vi "Group Publishing.vi"() -> ()   [LabVIEW 2020, in "VectoScratch.lvlib"]
uses:
  VectoScratch.lvlib
  Vecto/Group Info.ctl
  Vecto/Publish Config.ctl
  Vecto/Channel Init.ctl
  4d34a514-e5b9-4f11-b735-09902ffeac7b.vi
  Vecto/ChannelService/ChannelService.lvclass
  Vecto/RemoteDataService/RemoteDataService.lvclass
  Vecto/Vecto.lvlib
  Vecto/Group Config/Group Config.lvclass
  Vecto/Group/Group.lvclass
  Vecto/SequenceCountService/SequenceCountService.lvclass
panel:
  in  "Groups":i32=100
  in  "Rate":i32=10
  in  "Count":i32=150
  out "error out":errorcluster
  out "i":i32
  in  "stop":bool
  in  "Publish Address":string="230.0.0.100"
  in  "Publish Port":u16=20000
  in  "Node Name":string="Alpha"
  in  "Values":dbl[][](array[slide]) scale=0.0..1000.0
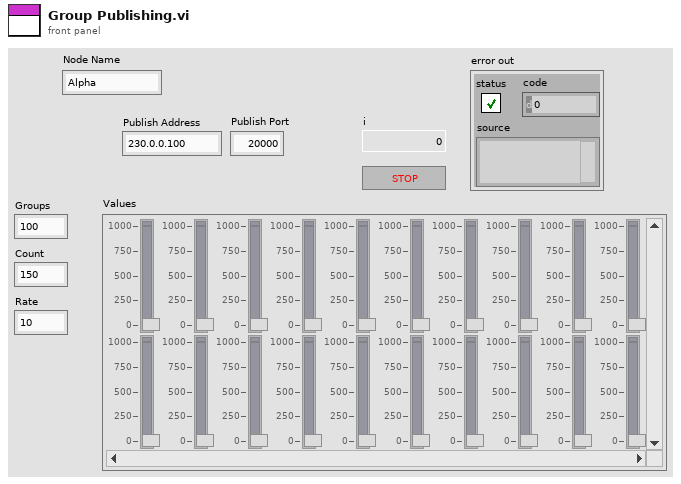
[diagram p1: front panel]
types:
  T1 = typedef "Vecto.lvlib/Publish Config.ctl" = cluster{"Address":string, "Port":u16}
  T2 = typedef "Vecto.lvlib/Group Info.ctl" = cluster{"System":string, "Cluster":string, "Node":string, "Task":string, "Name":string}
  T3 = typedef "Vecto.lvlib/Channel Init.ctl" = cluster{"Name":string, "Resource":string}
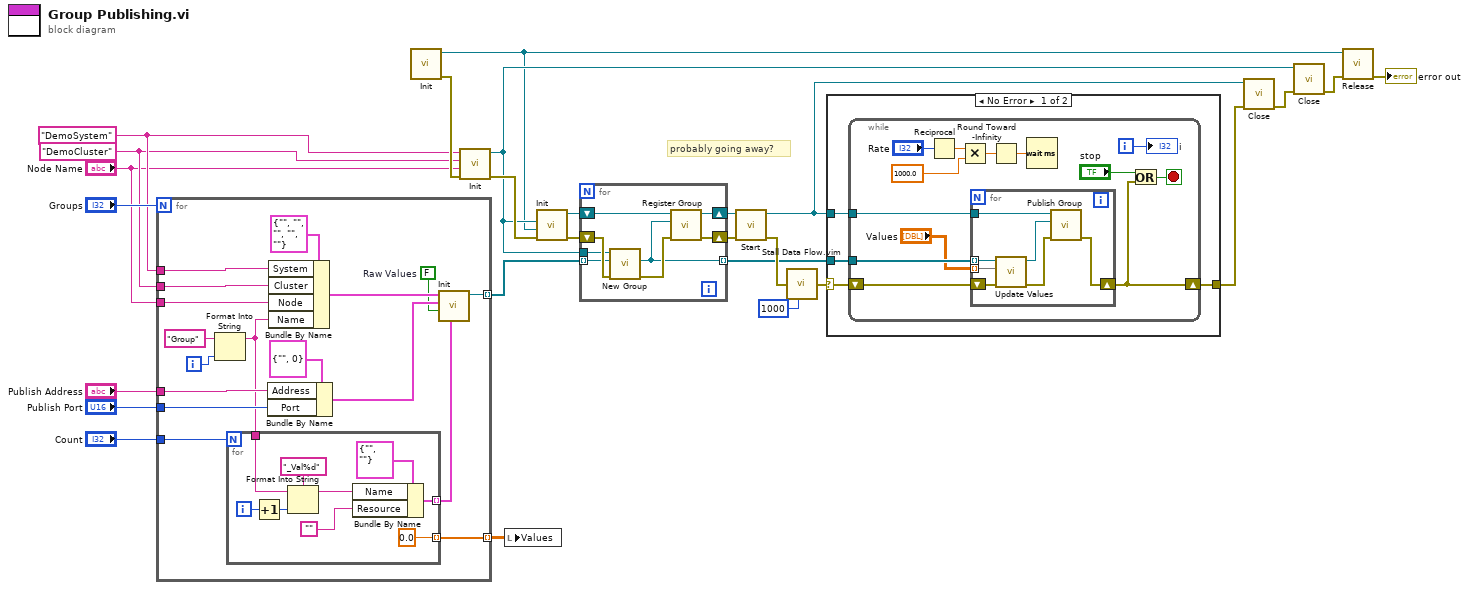
[diagram p0: block diagram]
diagram:
  w14 = "DemoSystem" ("System")
  w13 = "DemoCluster" ("Cluster")
  # "probably going away?"
  n1 = for {
    N: "Groups" -> [_]
    tunnel: w14 -> [w42]
    tunnel: w13 -> [w41]
    tunnel: "Node Name" -> [w40]
    tunnel: "Publish Address" -> [w38]
    tunnel: "Publish Port" -> [w37]
    tunnel: [w32] -> w21 mode=indexing
    tunnel: [w31] -> w20 mode=indexing
    tunnel: "Count" -> [w30]
    i -> [w28]
    w33 = FALSE  # Raw Values
    n2 = Format Into String(initial string="Group", w28) -> (resulting string=w27:string)  [unwired: 2 in, 1 out]
    n3 = for {
      N: w30 -> [_]
      tunnel: [w45] -> w34 mode=indexing
      tunnel: [0.0] -> w31 mode=indexing
      tunnel: w27 -> [w46]
      i -> [w52]
      n4 = Increment(x=w52) -> (x+1=w51:i32)
      n5 = Format Into String(format string="_Val%d", initial string=w46, w51) -> (resulting string=w49:string)  [unwired: 1 in, 1 out]
      n6 = Bundle By Name(cluster=T3 {"Name"="", "Resource"=""} ("Channel Init"), "Name"=w49, "Resource"="") -> (w45:T3)
    }
    n7 = Bundle By Name(cluster=T1 {"Address"="", "Port"=0} ("Publish Config"), "Address"=w38, "Port"=w37) -> (w35:T1)
    n8 = Bundle By Name(cluster=T2 {"System"="", "Cluster"="", "Node"="", "Task"="", "Name"=""} ("Group Info"), "System"=w42, "Cluster"=w41, "Node"=w40, "Name"=w27) -> (w36:T2)
    n9 = call "Init.vi"("Channels"=w34, "Raw Values (T)"=w33, "Publish Config (None)"=w35, "Group Info"=w36) -> ("Group Config out"=w32:refnum<class "Group Config.lvclass">)  [unwired: 6 in, 1 out]
  }
  n10 = call "Init.vi"() -> ("error out"=w24:errorcluster, "SequenceCountService out"=w2:refnum<class "SequenceCountService.lvclass">)  [unwired: 10 in]
  n11 = call "Init.vi"("error in (no error)"=w24, "Node"="Node Name", "Cluster"=w13, "System"=w14) -> ("error out"=w25:errorcluster, "ChannelService out"=w4:refnum<class "ChannelService.lvclass">)  [unwired: 6 in]
  n12 = local write "Values"(w20) -> ()
  n13 = call "Init.vi"("error in (no error)"=w25, "SequenceCountService"=w2, "ChannelService"=w4) -> ("error out"=w10:errorcluster, "RemoteDataService out"=w11:refnum<class "RemoteDataService.lvclass">)  [unwired: 7 in]
  n14 = for {
    tunnel: w4 -> [w58]
    tunnel: w21 -> [w54] mode=indexing
    tunnel: [w53] -> w17 mode=indexing
    shift-right: [w56] -> w9
    shift-left: w10 -> [w59]
    shift-right: [w55] -> w8
    shift-left: w11 -> [w57]
    n15 = call "New Group.vi"("error in (no error)"=w59, "Group Config"=w54, "ChannelService in"=w58) -> ("error out"=w60:errorcluster, "Group"=w53:refnum<class "Group.lvclass">)  [unwired: 6 in, 1 out]
    n16 = call "Register Group.vi"("error in (no error)"=w60, "Group"=w53, "RemoteDataService in"=w57) -> ("error out"=w56:errorcluster, "RemoteDataService out"=w55:refnum<class "RemoteDataService.lvclass">)  [unwired: 7 in]
  }
  n17 = call "Start.vi"("error in (no error)"=w9, "RemoteDataService in"=w8) -> ("error out"=w26:errorcluster, "RemoteDataService out"=w6:refnum<class "RemoteDataService.lvclass">)  [unwired: 8 in]
  n18 = call "Stall Data Flow.vim"("value in"=w26, "milliseconds to wait"=u32 1000) -> ("value out"=w16:errorcluster)  [unwired: 1 out]
  n19 = case shown="No Error" w16 {
    selector: w16 -> [w62 w85]
    tunnel: [w64 w85] -> w7
    tunnel: w17 -> [w63 _]
    tunnel: w6 -> [w61 _]
    frame No Error {
      n20 = while {
        shift-right: [w77] -> w64
        shift-left: w62 -> [w76]
        tunnel: w63 -> [w74]
        tunnel: w61 -> [w72]
        i -> [w71]
        stop <- w73 stop-if-true
        n21 = Reciprocal(x="Rate") -> (1/x=w69:dbl)
        n22 = Multiply(x=w69, y=1000.0) -> (x*y=w67:dbl)
        n23 = for {
          tunnel: w74 -> [w82] mode=indexing
          tunnel: w72 -> [w81]
          shift-right: [w84] -> w77
          shift-left: w76 -> [w83]
          tunnel: "Values" -> [w80] mode=indexing
          n24 = call "Update Values.vi"("error in (no error)"=w83, "Values"=w80, "Group in"=w82) -> ("error out"=w78:errorcluster, "Group out"=w79:refnum<class "Group.lvclass">)  [unwired: 7 in]
          n25 = call "Publish Group.vi"("error in (no error)"=w78, "Group"=w79, "RemoteDataService in"=w81) -> ("error out"=w84:errorcluster)  [unwired: 7 in, 1 out]
        }
        n26 = Round Toward -Infinity(1:w67) -> (0:w66:dbl)
        n27 = Wait (ms)(milliseconds to wait=w66) -> ()  [unwired: 1 out]
        n28 = Or(x="stop", y=w77) -> (x .or. y?=w73:bool)
        "i" <- w71
      }
    }
    frame Error {
    }
  }
  n29 = call "Close.vi"("error in (no error)"=w7, "RemoteDataService in"=w6) -> ("error out"=w5:errorcluster)  [unwired: 9 in]
  n30 = call "Close.vi"("error in (no error)"=w5, "ChannelService in"=w4) -> ("error out"=w3:errorcluster)  [unwired: 9 in]
  n31 = call "Release.vi"("error in (no error)"=w3, "SequenceCountService in"=w2) -> ("error out"=→"error out":errorcluster)  [unwired: 9 in]
